vi "MINDEO_Scanner.vi"(8 "error in (no error)":errorcluster, 11 "VISA resource name":refnum<visa-resource-name>) -> (0 "error out":errorcluster, 3 "trimmed string":string)   [LabVIEW 2011]
uses:
  <vilib>/Instr/_visa.llb/VISA Configure Serial Port (Instr).vi
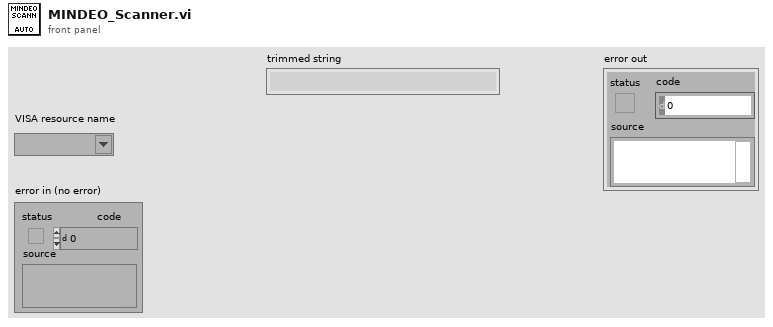
[diagram p1: front panel]
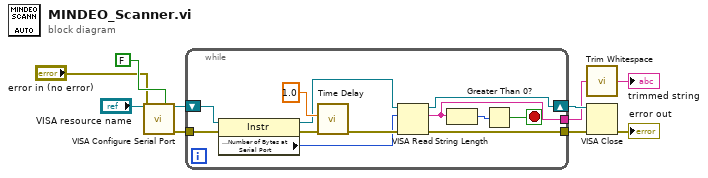
[diagram p0: block diagram]
diagram:
  n1 = call-poly "VISA Configure Serial Port"("VISA resource name"="VISA resource name", "Enable Termination\nChar (T)"=FALSE ("Enable Termination\nChar (T)"), "error in (no error)"="error in (no error)") -> ("VISA resource name out"=w7:refnum<visa-resource-name>, "error out"=w6:errorcluster)  [unwired: 11 in]
  n2 = while {
    tunnel: [w19] -> w4
    shift-right: [w20] -> w5
    shift-left: w7 -> [w16]
    tunnel: w6 -> [w15]
    tunnel: [w13] -> w3
    stop <- w11 stop-if-true
    n3 = property class="Instr"(reference=w16, error in=w15) -> (reference out=w17:refnum<visa-resource-name>, error out=w18:errorcluster, "Serial Settings:Number of Bytes at Serial Port"=w14:u32)
    n4 = call "Time Delay"("error in (no error)"=w18, "Delay Time (s)"=1.0) -> ("error out"=w21:errorcluster)  [unwired: 9 in]
    n5 = VISA Read(VISA resource name=w17, byte count=w14, error in (no error)=w21) -> (VISA resource name out=w20:refnum<visa-resource-name>, read buffer=w13:string, error out=w19:errorcluster)  [unwired: 1 out]
    n6 = String Length(string=w13) -> (length=w12:i32)
    n7 = Greater Than 0?(x=w12) -> (x > 0?=w11:bool)
  }
  n8 = call <vilib>:"Trim Whitespace.vi"("string"=w3) -> ("trimmed string"=→"trimmed string":string)  [unwired: 1 in]
  n9 = VISA Close(VISA resource name=w5, error in (no error)=w4) -> (error out=→"error out":errorcluster)
